vi "File.Build Path, Check for invalid Characters.vi"(9 "SubDir Name":string, 11 "Folder":path) -> (3 "New Path":path)   [LabVIEW 2018]
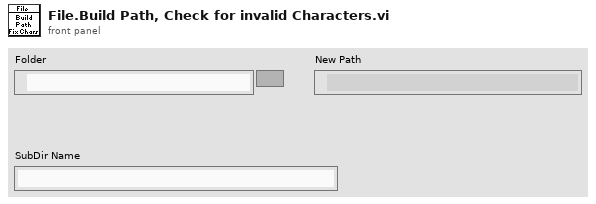
[diagram p1: front panel]
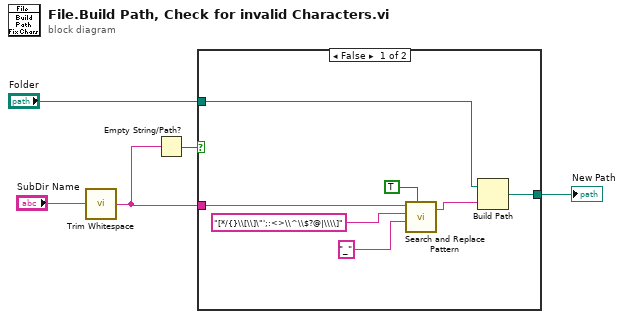
[diagram p0: block diagram]
diagram:
  n1 = call <vilib>:"Trim Whitespace.vi"("string"="SubDir Name") -> ("trimmed string"=w4:string)  [unwired: 1 in]
  n2 = Empty String/Path?(string/path=w4) -> (empty?=w1:bool)
  n3 = case shown="False" w1 {
    tunnel: w4 -> [w11 _]
    tunnel: [w7 w13] -> w3
    tunnel: "Folder" -> [w6 w13]
    frame False {
      n4 = call <vilib>:"Search and Replace Pattern.vi"("string"=w11, "regular expression (\"\")"="[*/{}\\[\\]\"';:<>\\^\\$?@|\\\\]" ("regular expression (\"\")"), "replace string (\"\")"="_" ("regular expression (\"\")"), "replace all? (F)"=TRUE) -> ("result string"=w8:string)  [unwired: 1 in, 1 out]
      n5 = Build Path(base path=w6, name or relative path=w8) -> (appended path=w7:path)
    }
    frame True {
    }
  }
  "New Path" <- w3
